vi "MetaServerSendStop.vi"() -> ()   [LabVIEW 2017]
panel:
  out "bytes written":i32
  in  "String To Send":string
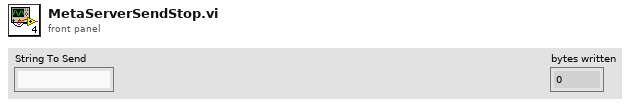
[diagram p1: front panel]
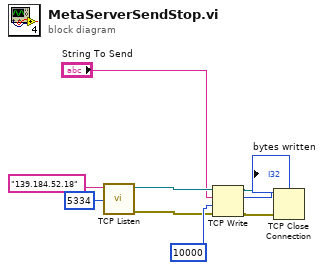
[diagram p0: block diagram]
diagram:
  n1 = call <vilib>:"TCP Listen.vi"("port"=u16 5334, "service name"="139.184.52.18" ("address")) -> ("error out"=w5:errorcluster, "connection ID"=w6:refnum<k5>)  [unwired: 5 in, 3 out]
  n2 = TCP Write(connection ID=w6, data in="String To Send", error in (no error)=w5, 9:10000 ("timeout ms (25000)")) -> (connection ID out=w9:refnum<k5>, bytes written=→"bytes written":i32, error out=w8:errorcluster)
  n3 = TCP Close Connection(connection ID=w9, error in (no error)=w8) -> ()  [unwired: 1 in, 2 out]
